vi "GetItemByPath.vi"(8 "error in (no error)":errorcluster, 9 "Path":string, 11 "CRuleList in":refnum<class "CRuleList.lvclass">) -> (0 "error out":errorcluster, 1 "IDependencyItemRule":refnum<class "IDependencyItemRule.lvclass">, 2 "key found?":bool, 3 "CRuleList out":refnum<class "CRuleList.lvclass">)   [LabVIEW 2020, in "DependencyInspection.lvlib" / "CRuleList.lvclass"]
uses:
  CRuleList.lvclass
  obj/Addons/LabVIEWObjectInterfaces.lvlibp/LabVIEWObjectInterfaces/IDependencyItemRule/IDependencyItemRule.lvclass
  CRuleList.lvclass/CRuleList.ctl
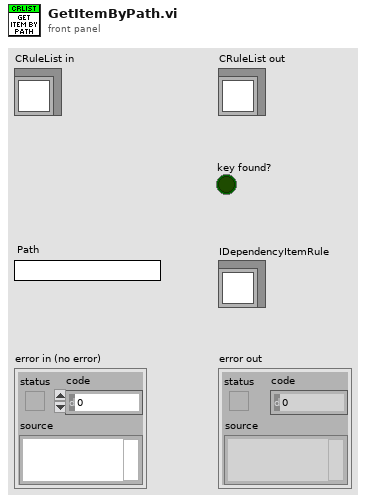
[diagram p1: front panel]
types:
  T1 = typedef "DependencyInspection.lvlib/CRuleList.lvclass/RuleListRef.ctl" = refnum<data-value>
  T2 = typedef "DependencyInspection.lvlib/CRuleList.lvclass/RuleList.ctl" = map{string, refnum<class "IDependencyItemRule.lvclass">}
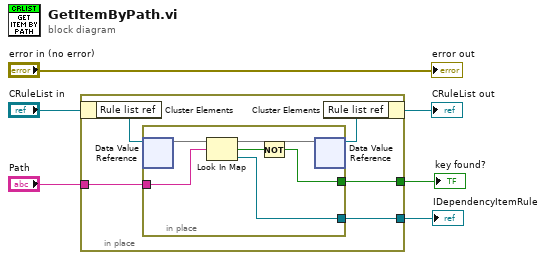
[diagram p0: block diagram]
diagram:
  n1 = in-place {
    in-place-border: "Path" -> [w11]
    in-place-border: [w10] -> w5
    in-place-border: [w9] -> w1
    n2 = in-place-cluster #1("CRuleList in") -> ("Rule list ref"=w8:T1)
    n3 = in-place {
      in-place-border: w11 -> [w16]
      in-place-border: [w15] -> w10
      in-place-border: [w14] -> w9
      n4 = in-place-dvr #2(w8) -> (w12:T2)  [unwired: 1 out]
      n5 = Look In Map(map=w12, key=w16) -> (key not found?=w13:bool, value=w14:refnum<class "IDependencyItemRule.lvclass">)  [unwired: 1 in]
      n6 = Not(x=w13) -> (.not. x?=w15:bool)
      n7 = in-place-dvr #2(w12) -> (w7:T1)  [unwired: 1 out]
    }
    n8 = in-place-cluster #1("Rule list ref"=w7) -> (→"CRuleList out":refnum<class "CRuleList.lvclass">)
  }
  "key found?" <- w5
  "IDependencyItemRule" <- w1
  "error out" <- "error in (no error)"
